vi "Elapsed Time.vi"(2 "second error in":errorcluster, 3 "first error in":errorcluster) -> (0 "ms time":u32)   [LabVIEW 2015]
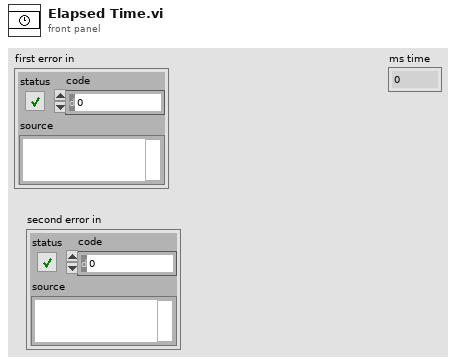
[diagram p1: front panel]
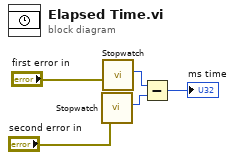
[diagram p0: block diagram]
diagram:
  n1 = call "Stopwatch.vi"("error in (no error)"="second error in") -> ("millisecond timer value"=w3:u32)  [unwired: 5 in, 1 out]
  n2 = call "Stopwatch.vi"("error in (no error)"="first error in") -> ("millisecond timer value"=w2:u32)  [unwired: 5 in, 1 out]
  n3 = Subtract(x=w2, y=w3) -> (x-y=→"ms time":u32)
